vi "Get Background Image JPG Path.vi"(3 "Inkscape Path":path) -> (1 "Background JPG Path":path)   [LabVIEW 2019]
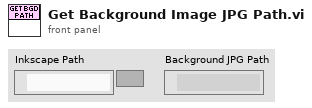
[diagram p1: front panel]
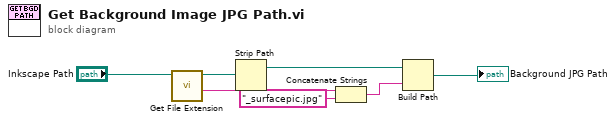
[diagram p0: block diagram]
diagram:
  n1 = call <vilib>:"Get File Extension.vi"("file"="Inkscape Path") -> ("filename without extension"=w5:string, "dup file"=w6:path)  [unwired: 6 in, 3 out]
  n2 = Strip Path(path=w6) -> (stripped path=w3:path)  [unwired: 1 out]
  n3 = Concatenate Strings(w5, "_surfacepic.jpg" ("string")) -> (w2:string)
  n4 = Build Path(base path=w3, name or relative path=w2) -> (appended path=→"Background JPG Path":path)
